vi "Algorithms.vi"() -> ()   [LabVIEW 2013]
uses:
  globals.vi
  qwtblvlib/QWTBLVLib.lvlib
panel:
  in  "hide this panel":bool
  in  "details":bool
  out "Outputs descriptions":string
  out "Inputs descriptions":string
  out "Required Inputs":string
  out "Optional Inputs":string
  out "Provides MCM":bool
  out "Provides GUF":bool
  out "License":string
  out "Remarks":string
  out "Citation":string
  out "Description":string
  out "Name":string
  in  "curAlg":u16(ring) caption="Selected Algorithm ID" items=["ADEV", "CCC", "FPNLSF", "FourPSF", "INL-DNL", "MADEV", "OADEV", "PSFE"]
  in  "reload alginfo":bool
  # "Algorithm"
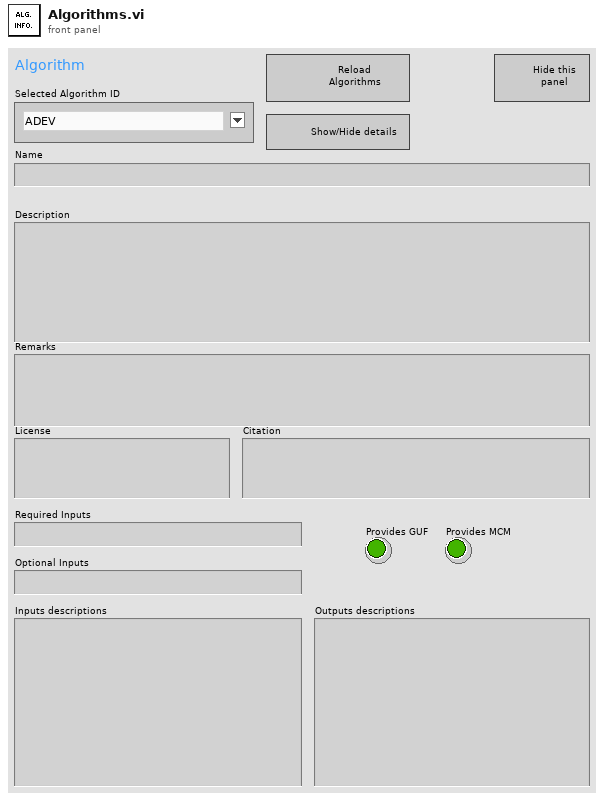
[diagram p1: front panel]
types:
  T1 = typedef "LVRectTypeDef.ctl" = cluster{"Left":i16, "Top":i16, "Right":i16, "Bottom":i16}
  T2 = typedef "QWTBLVLib.lvlib/TD Algorithm Information.ctl" = cluster{"ID":string, "Name":string, "Description":string, "Citation":string, "Remarks":string, "License":string, "Inputs":T3[], "Outputs":T4[], "Provides GUF":bool, "Provides MCM":bool, "Full path":string}
  T3 = typedef "QWTBLVLib.lvlib/TD Algorithm Information Input.ctl" = cluster{"Name":string, "Description":string, "Alternative":i32, "Optional":i32, "Parameter":i32}
  T4 = typedef "QWTBLVLib.lvlib/TD Algorithm Information Output.ctl" = cluster{"Name":string, "Description":string}
  T5 = enum32{"Invalid", "Standard", "Closed", "Hidden", "Minimized", "Maximized"}
  T6 = typedef "TD GUI Settings.ctl" = cluster{"Backend engine":T7, "QWTB Folder Path":path}
  T7 = typedef "QWTBLVLib.lvlib/TD Backend Engine.ctl" = enum16{"Matlab by Script node", "GNU Octave by GOLPI"}
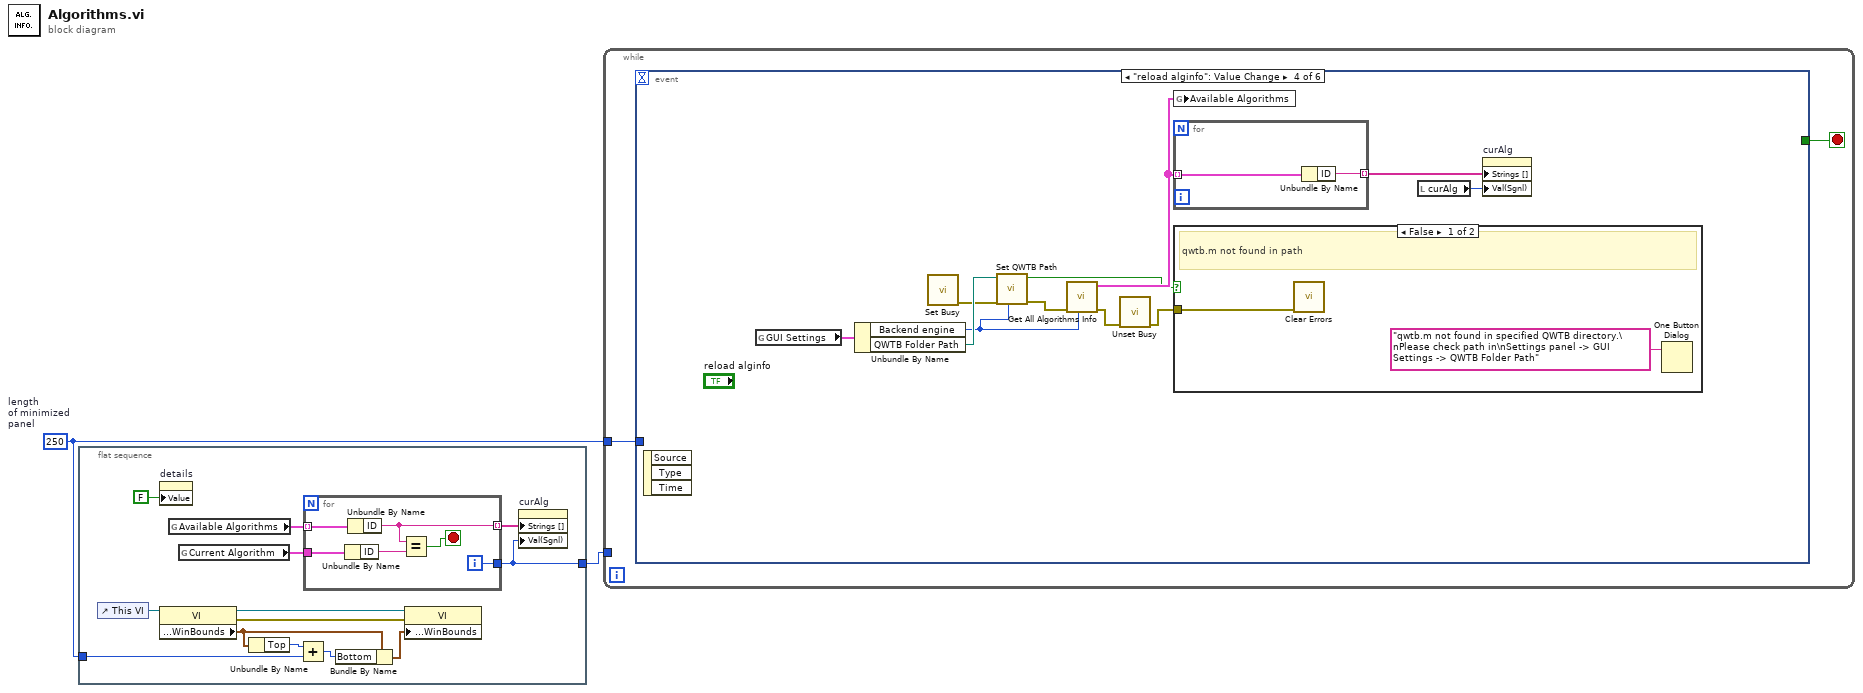
[diagram p0: block diagram]
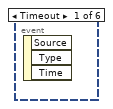
[diagram p2: hidden frame]
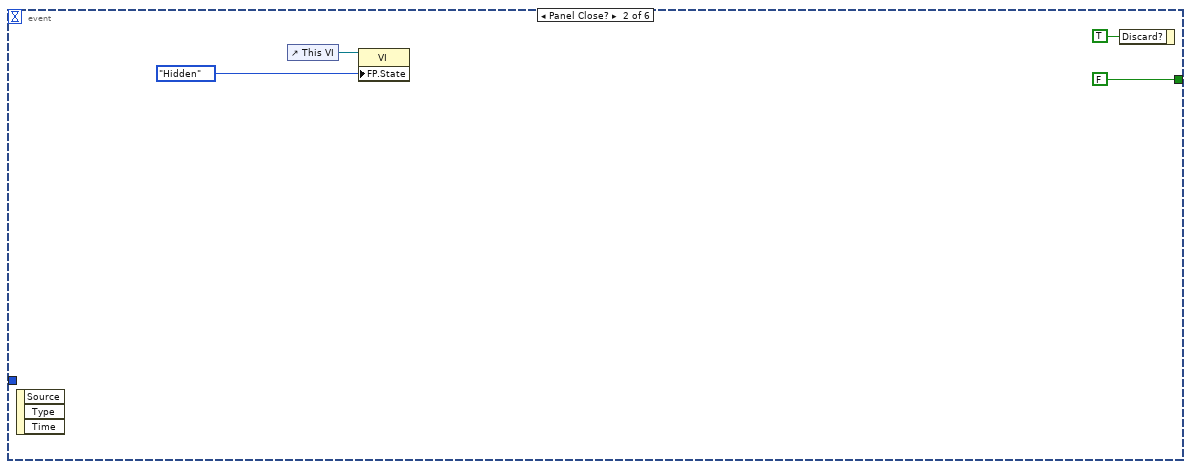
[diagram p3: hidden frame]
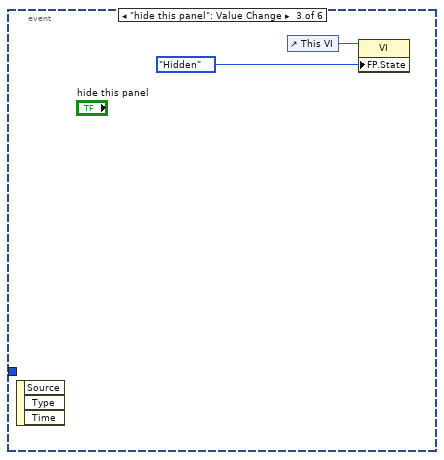
[diagram p4: hidden frame]
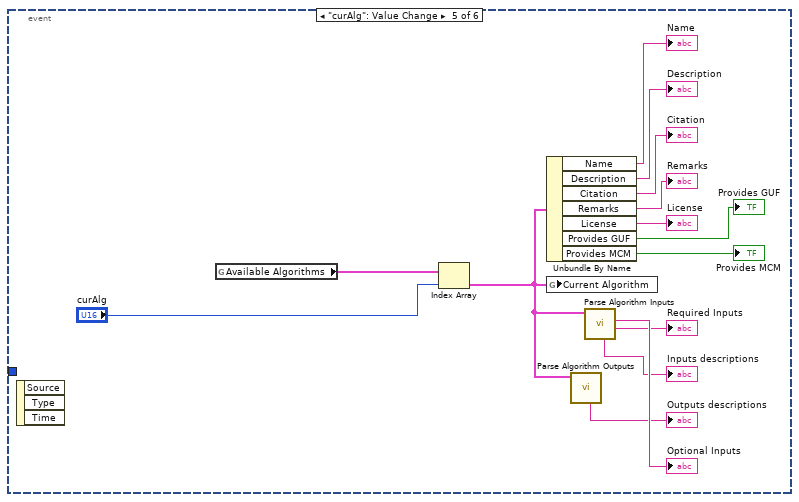
[diagram p6: hidden frame]
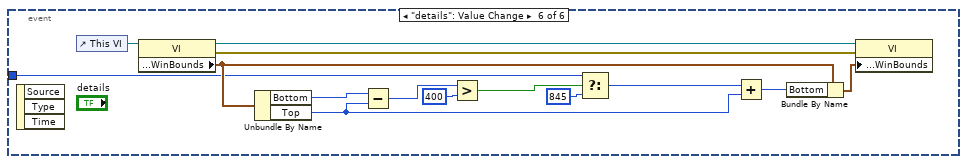
[diagram p7: hidden frame]
diagram:
  w1 = i16 250  # length of minimized panel
  n1 = flat-sequence {
    tunnel: [w13] -> w2
    tunnel: w1 -> [w3]
    frame #0 {
      n2 = control-ref of="This VI"() -> (w7:refnum<vi>)
      n3 = property on="details" class="Bool (strict)"("Value"=FALSE ("details")) -> ()  [unwired: 2 in, 2 out]
      n4 = property class="VI"(reference=w7) -> (reference out=w8:refnum<vi>, error out=w10:errorcluster, "Front Panel.WinBounds"=w6:T1)  [unwired: 1 in]
      n5 = global read "globals.vi" "Available Algorithms"() -> (w14:T2[])
      n6 = global read "globals.vi" "Current Algorithm"() -> (w15:T2)
      n7 = Unbundle By Name(w6) -> ("Top"=w5:i16)
      n8 = Add(x=w5, y=w3) -> (x+y=w4:i16)
      n9 = for {
        tunnel: w15 -> [w20]
        tunnel: w14 -> [w21] mode=indexing
        tunnel: [w17] -> w13
        tunnel: [w16] -> w12 mode=indexing
        i -> [w17]
        stop <- w18 stop-if-true
        n10 = Unbundle By Name(w20) -> ("ID"=w19:string)
        n11 = Unbundle By Name(w21) -> ("ID"=w16:string)
        n12 = Equal?(x=w16, y=w19) -> (x = y?=w18:bool)
      }
      n13 = Bundle By Name(cluster=w6, "Bottom"=w4) -> (w9:T1)
      n14 = property class="VI"(reference=w8, error in=w10, "Front Panel.WinBounds"=w9) -> ()  [unwired: 2 out]
      n15 = property on="curAlg" class="Ring (strict)"("Strings []"=w12, "Val(Sgnl)"=w13) -> ()  [unwired: 2 in, 2 out]
    }
  }
  n16 = while {
    tunnel: w2 -> [_]
    tunnel: w1 -> [w22]
    stop <- w23 stop-if-true
    n17 = event shown="[3] \"reload alginfo\": Value Change" {
      selector: _ -> [_ _ _ _ _ _]
      dyn-events: _ -> [_ _ _ _ _ _]
      timeout: _ -> [_ _ _ _ _ _]
      tunnel: [_ FALSE ("cancel") _ _ _ _] -> w23
      tunnel: w22 -> [_ _ _ _ _ w59]
      event Timeout {
        n18 = event-data() -> ()  [unwired: 1 in, 3 out]
      }
      event Panel Close? {
        n19 = event-data() -> ()  [unwired: 1 in, 3 out]
        n20 = control-ref of="This VI"() -> (w26:refnum<vi>)
        n21 = property class="VI"(reference=w26, "FP.State"=T5."Hidden" ("Front Panel Window:State")) -> ()  [unwired: 1 in, 2 out]
        n22 = event-data("Discard?"=TRUE) -> ()  [unwired: 1 in, 1 out]
      }
      event "hide this panel": Value Change {
        n23 = event-data() -> ()  [unwired: 1 in, 3 out]
        n24 = control-ref of="This VI"() -> (w29:refnum<vi>)
        n25 = property class="VI"(reference=w29, "FP.State"=T5."Hidden" ("Front Panel Window:State")) -> ()  [unwired: 1 in, 2 out]
      }
      event "reload alginfo": Value Change {
        n26 = event-data() -> ()  [unwired: 1 in, 3 out]
        n27 = global read "globals.vi" "GUI Settings"() -> (w37:T6)
        n28 = Unbundle By Name(w37) -> ("Backend engine"=w34:T7, "QWTB Folder Path"=w36:path)
        n29 = call <vilib>:"Set Busy.vi"() -> ("error out"=w32:errorcluster)  [unwired: 10 in, 1 out]
        n30 = call "Set QWTB Path.vi"("Backend engine"=w34, "error in"=w32, "QWTB Folder Path"=w36) -> ("error out"=w35:errorcluster, "qwtb.m found in path"=w33:bool)  [unwired: 7 in]
        n31 = call "Get All Algorithms Info.vi"("Backend engine"=w34, "error in"=w35) -> ("error out"=w31:errorcluster, "All Algorithms Info"=w40:T2[])  [unwired: 8 in]
        n32 = call <vilib>:"Unset Busy.vi"("error in (no error)"=w31) -> ("error out"=w30:errorcluster)  [unwired: 10 in]
        n33 = global write "globals.vi" "Available Algorithms"(w40) -> ()
        n34 = for {
          tunnel: w40 -> [w44] mode=indexing
          tunnel: [w43] -> w38 mode=indexing
          n35 = Unbundle By Name(w44) -> ("ID"=w43:string)
        }
        n36 = case shown="False" w33 {
          tunnel: w30 -> [w41 _]
          frame False {
            # "qwtb.m not found in path"
            n37 = call <vilib>:"Clear Errors.vi"("error in (no error)"=w41) -> ()  [unwired: 6 in, 1 out]
            n38 = One Button Dialog(message="qwtb.m not found in specified QWTB directory.\nPlease check path in\nSettings panel -> GUI Settings -> QWTB Folder Path") -> ()  [unwired: 1 in, 1 out]
          }
          frame True {
          }
        }
        n39 = local read "curAlg"() -> (w39:u16)
        n40 = property on="curAlg" class="Ring (strict)"("Strings []"=w38, "Val(Sgnl)"=w39) -> ()  [unwired: 2 in, 2 out]
      }
      event "curAlg": Value Change {
        n41 = event-data() -> ()  [unwired: 1 in, 3 out]
        n42 = global read "globals.vi" "Available Algorithms"() -> (w58:T2[])
        n43 = Index Array(array=w58, index="curAlg") -> (element=w46:T2)
        n44 = Unbundle By Name(w46) -> ("Name"=→"Name":string, "Description"=→"Description":string, "Citation"=→"Citation":string, "Remarks"=→"Remarks":string, "License"=→"License":string, "Provides GUF"=→"Provides GUF":bool, "Provides MCM"=→"Provides MCM":bool)
        n45 = global write "globals.vi" "Current Algorithm"(w46) -> ()
        n46 = call "Parse Algorithm Outputs.vi"("Algorithm Information"=w46) -> ("Q descriptions"=→"Outputs descriptions":string)  [unwired: 9 in, 1 out]
        n47 = call "Parse Algorithm Inputs.vi"("Algorithm Information"=w46) -> ("Required Q as string"=→"Required Inputs":string, "Optional Q as string"=→"Optional Inputs":string, "Q descriptions"=→"Inputs descriptions":string)  [unwired: 6 in, 2 out]
      }
      event "details": Value Change {
        n48 = event-data() -> ()  [unwired: 1 in, 3 out]
        n49 = control-ref of="This VI"() -> (w72:refnum<vi>)
        n50 = property class="VI"(reference=w72) -> (reference out=w67:refnum<vi>, error out=w65:errorcluster, "Front Panel.WinBounds"=w68:T1)  [unwired: 1 in]
        n51 = Unbundle By Name(w68) -> ("Bottom"=w64:i16, "Top"=w61:i16)
        n52 = Subtract(x=w64, y=w61) -> (x-y=w63:i16)
        n53 = Greater?(x=w63, y=i16 400) -> (0:w70:bool)
        n54 = Select(t=w59, s=w70, f=i16 845 ("y")) -> (s? t:f=w62:i16)
        n55 = Add(x=w62, y=w61) -> (x+y=w60:i16)
        n56 = Bundle By Name(cluster=w68, "Bottom"=w60) -> (w66:T1)
        n57 = property class="VI"(reference=w67, error in=w65, "Front Panel.WinBounds"=w66) -> ()  [unwired: 2 out]
      }
    }
  }
